vi ".NET File Dialog.vi"(7 "Dialog Message":string, 8 "Error In":errorcluster, 11 "Initial Folder Path":path) -> (0 "Error Out":errorcluster, 1 "Cancelled?":bool, 2 "File Exist?":bool[](array[boolean]), 3 "File Path Array":path[](array[path]))   [LabVIEW 2021, in "Files.lvlib"]
uses:
  Files.lvlib
  System.Windows.Forms
panel:
  in  "Multiselect (F)":bool
  in  "File Filter List":string
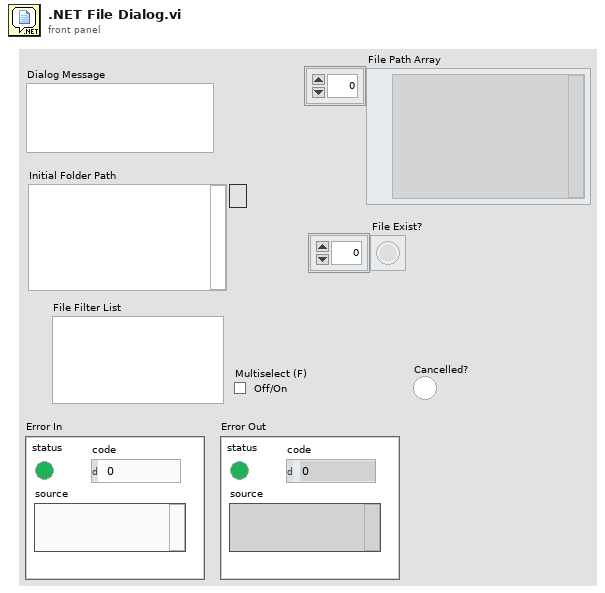
[diagram p1: front panel]
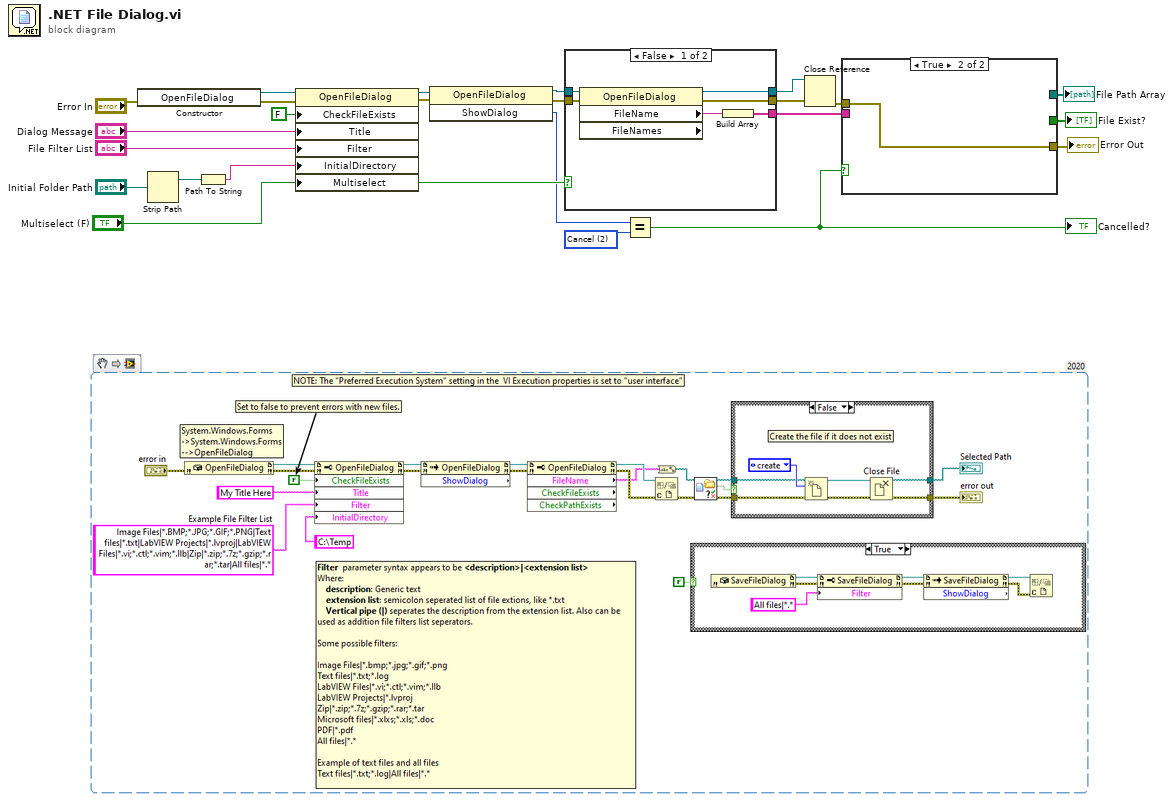
[diagram p0: block diagram]
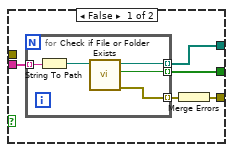
[diagram p2: hidden frame]
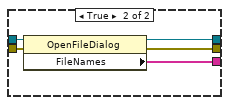
[diagram p3: hidden frame]
diagram:
  w3 = 2 items=["None", "OK", "Cancel", "Abort", "Retry", "Ignore", "Yes", "No"] ("ShowDialog")
  n1 = constructor class="OpenFileDialog"(error in="Error In") -> (reference out=w23:refnum<k24>, error out=w21:errorcluster)  [unwired: 2 in, 1 out]
  n2 = Strip Path(path="Initial Folder Path") -> (stripped path=w17:path)  [unwired: 1 out]
  n3 = Path To String(path=w17) -> (string=w16:string)
  n4 = property class="OpenFileDialog"(reference=w23, error in=w21, "CheckFileExists"=FALSE, "Title"="Dialog Message", "Filter"="File Filter List", "InitialDirectory"=w16, "Multiselect"="Multiselect (F)") -> (reference out=w15:refnum<k24>, error out=w14:errorcluster)
  n5 = invoke class="OpenFileDialog" method="ShowDialog"(reference=w15, error in=w14) -> (reference out=w13:refnum<k24>, error out=w11:errorcluster, "ShowDialog"=w4:i32)  [unwired: 1 in]
  n6 = case shown="False" "Multiselect (F)" {
    tunnel: w13 -> [w30 w35]
    tunnel: w11 -> [w29 w34]
    tunnel: [w27 w33] -> w8
    tunnel: [w26 w31] -> w10
    tunnel: [w25 w32] -> w9
    frame False {
      n7 = property class="OpenFileDialog" props=["FileName", "FileNames"](reference=w30, error in=w29) -> (reference out=w25:refnum<k24>, error out=w26:errorcluster, "FileName"=w28:string)  [unwired: 1 out]
      n8 = Build Array(w28) -> (w27:string[])
    }
    frame True {
      n9 = property class="OpenFileDialog"(reference=w35, error in=w34) -> (reference out=w32:refnum<k24>, error out=w31:errorcluster, "FileNames"=w33:string[])
    }
  }
  n10 = Equal?(x=w4, y=w3) -> (x = y?=w2:bool)
  "Cancelled?" <- w2
  n11 = Close Reference(reference=w9, error in (no error)=w10) -> (error out=w1:errorcluster)
  n12 = case shown="True" w2 {
    tunnel: w8 -> [w40 _]
    tunnel: [w39 _] -> w7
    tunnel: [w38 _] -> w6
    tunnel: [w36 w46] -> w5
    tunnel: w1 -> [_ w46]
    frame False {
      n13 = for {
        tunnel: w40 -> [w45] mode=indexing
        tunnel: [w43] -> w39 mode=indexing
        tunnel: [w42] -> w38 mode=indexing
        tunnel: [w41] -> w37 mode=indexing
        n14 = String To Path(string=w45) -> (path=w44:path)
        n15 = call <vilib>:"Check if File or Folder Exists.vi"("path"=w44) -> ("error out"=w41:errorcluster, "file or folder exists?"=w42:bool, "dup path"=w43:path)  [unwired: 8 in]
      }
      n16 = Merge Errors(w37) -> (w36:errorcluster)
    }
    frame True {
    }
  }
  "Error Out" <- w5
  "File Path Array" <- w7
  "File Exist?" <- w6
